vi "Fetch Min Max Waveform.vi"(7 "Waveform Start (1)":i32=1, 8 "error in (no error)":errorcluster {"code" format="%.0x"}, 9 "Waveform End (10000)":i32=10000, 10 "Source (\"CH1\")":string(combo)="CH1", 11 "VISA Resource Name":refnum<visa-resource-name>) -> (0 "error out":errorcluster {"code" format="%.0x"}, 1 "X Increment":dbl format="%.2e", 2 "Initial X":dbl format="%.2e", 3 "VISA Resource Name Out":refnum<visa-resource-name>, 4 "Max Waveform Array":dbl[](array[numeric]) format="%.2f", 5 "Actual Points":u32, 6 "Min Waveform Array":dbl[](array[numeric]) format="%.2f")   [LabVIEW 2010, in "Tektronix TDS 3000 Series.lvlib"]
doc: "This VI reads the current min max waveform (starting and ending at Waveform Start and Waveform End,respectively) from the oscilloscope, scales the data, and returns an array of DBLs. To obtain the complete waveform, use the default values on the waveform start and waveform end controls.\n\nNote:\n(1) In order for this VI to work the waveform must be displayed on the instrument.\n(2) This is only used with Normal and Average Acquisition Types\n(3) The instrument will return an error if you attempt to read more points than stored on the instrument. Set the desired record length in the Configure Acquisition Record VI."
uses:
  <instrlib>/Tektronix TDS 3000 Series/Tektronix TDS 3000 Series.lvlib
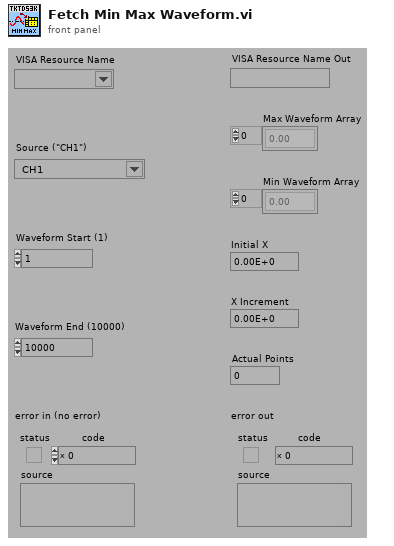
[diagram p1: front panel]
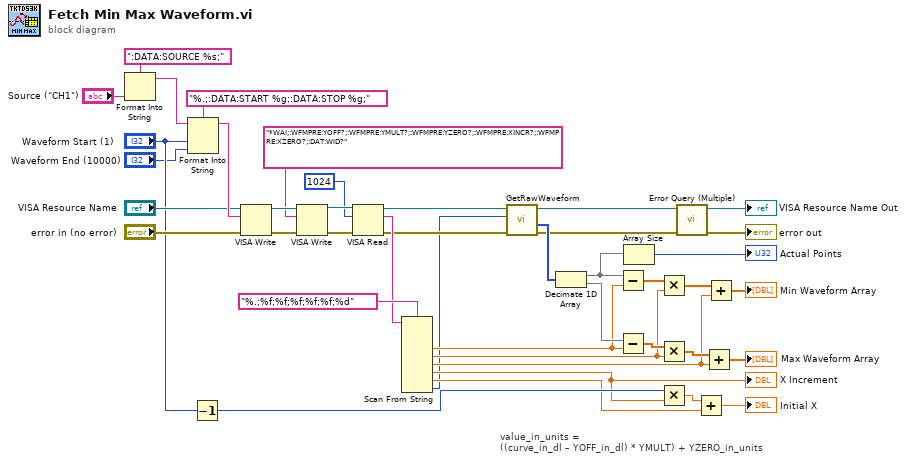
[diagram p0: block diagram]
diagram:
  # "value_in_units =\n((curve_in_dl – YOFF_in_dl) * YMULT) + YZERO_in_units"
  n1 = Format Into String(format string=":DATA:SOURCE %s;", "Source (\"CH1\")") -> (resulting string=w33:string)  [unwired: 2 in, 1 out]
  n2 = Format Into String(format string="%.;:DATA:START %g;:DATA:STOP %g;", initial string=w33, "Waveform Start (1)", "Waveform End (10000)") -> (resulting string=w36:string)  [unwired: 1 in, 1 out]
  n3 = Decrement(x="Waveform Start (1)") -> (x-1=w28:i32)
  n4 = VISA Write(VISA resource name="VISA Resource Name", write buffer=w36, error in (no error)="error in (no error)") -> (VISA resource name out=w38:refnum<visa-resource-name>, error out=w37:errorcluster)  [unwired: 1 out]
  n5 = VISA Write(VISA resource name=w38, write buffer="*WAI;:WFMPRE:YOFF?;:WFMPRE:YMULT?;:WFMPRE:YZERO?;:WFMPRE:XINCR?;:WFMPRE:XZERO?;:DAT:WID?", error in (no error)=w37) -> (VISA resource name out=w39:refnum<visa-resource-name>, error out=w40:errorcluster)  [unwired: 1 out]
  n6 = VISA Read(VISA resource name=w39, byte count=u32 1024 ("byte count (0)"), error in (no error)=w40) -> (VISA resource name out=w7:refnum<visa-resource-name>, read buffer=w22:string, error out=w6:errorcluster)  [unwired: 1 out]
  n7 = Scan From String(format string="%.;%f;%f;%f;%f;%f;%d", input string=w22) -> (output 1=w18:dbl, output 2=w17:dbl, output 3=w16:dbl, output 4=w23:dbl, output 5=w26:dbl, output 6=w5:i32)  [unwired: 8 in, 3 out]
  "X Increment" <- w23
  n8 = call <instrlib>:"GetRawWaveform.vi"("error in (no error)"=w6, "Byte Size per point (1 byte)"=w5, "VISA Resource Name"=w7) -> ("error out"=w3:errorcluster, "Waveform Array"=w32:i16[], "VISA Resource Name Out"=w4:refnum<visa-resource-name>)  [unwired: 6 in]
  n9 = Decimate 1D Array(w32) -> (w9:i16[], w19:i16[])
  n10 = Subtract(x=w9, y=w18) -> (x-y=w21:dbl[])
  n11 = Subtract(x=w19, y=w18) -> (x-y=w29:dbl[])
  n12 = Array Size(array=w9) -> (size(s)=→"Actual Points":i32)
  n13 = Multiply(x=w21, y=w17) -> (x*y=w20:dbl[])
  n14 = Multiply(x=w29, y=w17) -> (x*y=w30:dbl[])
  n15 = Multiply(x=w28, y=w23) -> (x*y=w27:dbl)
  n16 = call <instrlib>:"Error Query (Multiple).vi"("error in (no error)"=w3, "VISA Resource Name"=w4) -> ("error out"=→"error out":errorcluster, "VISA Resource Name Out"=→"VISA Resource Name Out":refnum<visa-resource-name>)  [unwired: 6 in, 2 out]
  n17 = Add(x=w27, y=w26) -> (x+y=→"Initial X":dbl)
  n18 = Add(x=w30, y=w16) -> (x+y=→"Max Waveform Array":dbl[])
  n19 = Add(x=w20, y=w16) -> (x+y=→"Min Waveform Array":dbl[])
